vi "Init.vi"(8 "error in (no error)":errorcluster, 10 "Camera ID":string, 11 "ZWO_ASI in":refnum<class "ZWO_ASI.lvclass">) -> (0 "error out":errorcluster, 3 "ZWO_ASI out":refnum<class "ZWO_ASI.lvclass">)   [LabVIEW 2023, in "ZWO_ASI.lvlib" / "ZWO_ASI.lvclass"]
uses:
  ZWO_ASI.lvclass
  ZWO_ASI.lvclass/ZWO_ASI.ctl
  <userlib>/ASICamera2_no_err/ASICamera2_no_err.lvlib
  Interfaces/InitDeinitInterface/InitDeinitComm Messages/InitDone Msg/InitDone Msg.lvclass
  <vilib>/ActorFramework/Actor/Actor.lvclass
  typedefs/instrumentType.ctl
  typedefs/typedefs.lvlib
  Applications/National Instruments/LabVIEW 2023 64-bit/vi.lib/ActorFramework/Actor/Actor.lvclass
  Users/alexandrosspiliotis/Documents/LV_DAQ_Project/ConcreteClasses/ConcreteInstrumentClasses/CameraClasses/ZWO_ASI_LV/ZWO_ASI/ZWO_ASI.lvclass
  Users/alexandrosspiliotis/Documents/LV_DAQ_Project/Interfaces/AbstractInstrumentClasses/Cameras_LV/CameraInterface/CameraInterface.lvclass
  Users/alexandrosspiliotis/Documents/LV_DAQ_Project/Interfaces/InitDeinitInterface/InitDeinit/InitDeinit.lvclass
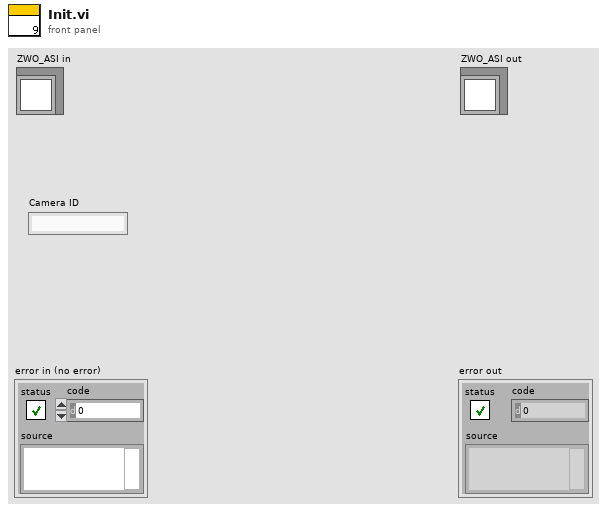
[diagram p1: front panel]
types:
  T1 = typedef "typedefs.lvlib/instrumentType.ctl" = enum16{"Spectrometer", "Camera", "Stepper"}
  T2 = cluster{"Name[0]":i8, "Name[1]":i8, "Name[2]":i8, "Name[3]":i8, "Name[4]":i8, "Name[5]":i8, "Name[6]":i8, "Name[7]":i8, "Name[8]":i8, "Name[9]":i8, "Name[10]":i8, "Name[11]":i8, "Name[12]":i8, "Name[13]":i8, "Name[14]":i8, "Name[15]":i8, "Name[16]":i8, "Name[17]":i8, "Name[18]":i8, "Name[19]":i8, "Name[20]":i8, "Name[21]":i8, "Name[22]":i8, "Name[23]":i8, "Name[24]":i8, "Name[25]":i8, "Name[26]":i8, "Name[27]":i8, "Name[28]":i8, "Name[29]":i8, "Name[30]":i8, "Name[31]":i8, "Name[32]":i8, "Name[33]":i8, "Name[34]":i8, "Name[35]":i8, "Name[36]":i8, "Name[37]":i8, "Name[38]":i8, "Name[39]":i8, "Name[40]":i8, "Name[41]":i8, "Name[42]":i8, "Name[43]":i8, "Name[44]":i8, "Name[45]":i8, "Name[46]":i8, "Name[47]":i8, "Name[48]":i8, "Name[49]":i8, "Name[50]":i8, "Name[51]":i8, "Name[52]":i8, "Name[53]":i8, "Name[54]":i8, "Name[55]":i8, "Name[56]":i8, "Name[57]":i8, "Name[58]":i8, "Name[59]":i8, "Name[60]":i8, "Name[61]":i8, "Name[62]":i8, "Name[63]":i8, "CameraID":i32, "MaxHeight":i32, "MaxWidth":i32, "IsColorCam":u32, "BayerPattern":u32, "SupportedBins[0]":i32, "SupportedBins[1]":i32, "SupportedBins[2]":i32, "SupportedBins[3]":i32, "SupportedBins[4]":i32, "SupportedBins[5]":i32, "SupportedBins[6]":i32, "SupportedBins[7]":i32, "SupportedBins[8]":i32, "SupportedBins[9]":i32, "SupportedBins[10]":i32, "SupportedBins[11]":i32, "SupportedBins[12]":i32, "SupportedBins[13]":i32, "SupportedBins[14]":i32, "SupportedBins[15]":i32, "SupportedVideoFormat[0]":u32, "SupportedVideoFormat[1]":u32, "SupportedVideoFormat[2]":u32, "SupportedVideoFormat[3]":u32, "SupportedVideoFormat[4]":u32, "SupportedVideoFormat[5]":u32, "SupportedVideoFormat[6]":u32, "SupportedVideoFormat[7]":u32, "@dummy control@":i8, "@dummy control@":i8, "@dummy control@":i8, "@dummy control@":i8, "PixelSize":dbl, "MechanicalShutter":u32, "ST4Port":u32, "IsCoolerCam":u32, "IsUSB3Host":u32, "IsUSB3Camera":u32, "ElecPerADU":sgl, "Unused[0]":i8, "Unused[1]":i8, "Unused[2]":i8, "Unused[3]":i8, "Unused[4]":i8, "Unused[5]":i8, "Unused[6]":i8, "Unused[7]":i8, "Unused[8]":i8, "Unused[9]":i8, "Unused[10]":i8, "Unused[11]":i8, "Unused[12]":i8, "Unused[13]":i8, "Unused[14]":i8, "Unused[15]":i8, "Unused[16]":i8, "Unused[17]":i8, "Unused[18]":i8, "Unused[19]":i8, "Unused[20]":i8, "Unused[21]":i8, "Unused[22]":i8, "Unused[23]":i8}
  T3 = typedef "typedefs.lvlib/InstrumentData.ctl" = cluster{"Instr Error":errorcluster, "Address":cluster{"address type":enum16{"VISA", "Index"}, "Address":string, "instrument type":T1}, "CurrentState":cluster{"Initialized":bool, "Connected":bool, "Running":bool, "Error":bool}, "Enqueuer":refnum<class "Message Enqueuer.lvclass">}
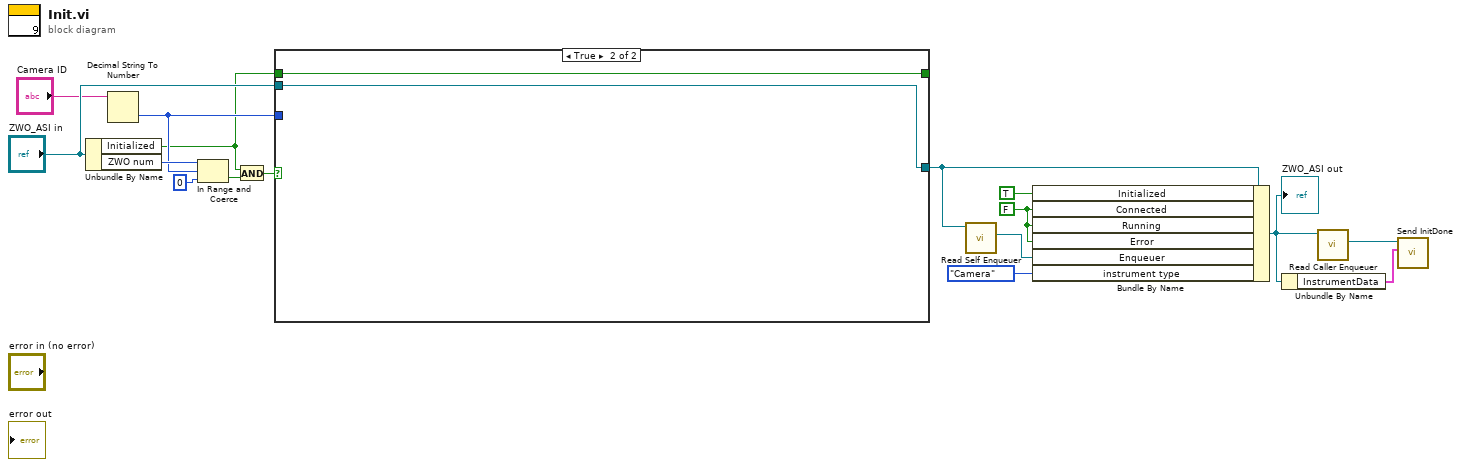
[diagram p0: block diagram]
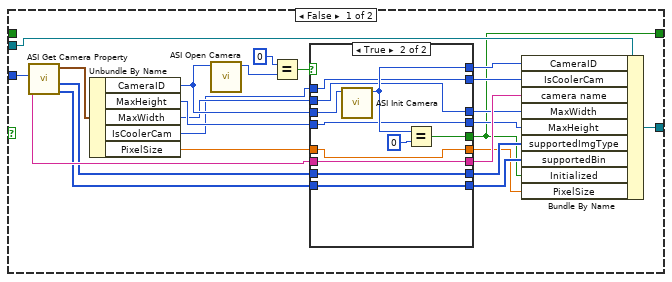
[diagram p2: hidden frame]
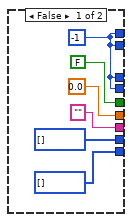
[diagram p3: hidden frame]
diagram:
  w6 = FALSE ("InstrumentData.CurrentState.Connected")
  n1 = Unbundle By Name("ZWO_ASI in") -> ("Initialized"=w8:bool, "ZWO num"=w14:i32)
  n2 = Decimal String To Number(string="Camera ID") -> (number=w10:i32)  [unwired: 2 in, 1 out]
  n3 = In Range and Coerce(upper limit=w14, x=w10, lower limit=0) -> (In Range?=w12:bool)  [unwired: 1 out]
  n4 = And(x=w8, y=w12) -> (x .and. y?=w11:bool)
  n5 = case shown="True" w11 {
    tunnel: w10 -> [w35 _]
    tunnel: "ZWO_ASI in" -> [w34 w58]
    tunnel: [w18 w59] -> _
    tunnel: w8 -> [_ w59]
    tunnel: [w17 w58] -> w2
    frame False {
      n6 = call <userlib>:"ASI Get Camera Property.vi"("iCameraIndex"=w35) -> ("supportedBin"=w27:i8[], "supportedImgType"=w26:i8[], "pASICameraInfo out"=w38:T2, "cameraName"=w31:string)  [unwired: 6 in, 1 out]
      n7 = Unbundle By Name(w38) -> ("CameraID"=w36:i32, "MaxHeight"=w29:i32, "MaxWidth"=w22:i32, "IsCoolerCam"=w21:u32, "PixelSize"=w20:dbl)
      n8 = call <userlib>:"ASI Open Camera.vi"("iCameraID"=w36) -> ("function return"=w40:i32)  [unwired: 10 in]
      n9 = Equal?(x=0, y=w40) -> (x = y?=w37:bool)
      n10 = case shown="True" w37 {
        tunnel: [FALSE w56] -> w18
        tunnel: w36 -> [_ w55]
        tunnel: [w45 w54] -> w33
        tunnel: [w45 w48] -> w32
        tunnel: w31 -> [_ w53]
        tunnel: ["" ("cameraName") w53] -> w30
        tunnel: w29 -> [_ w50]
        tunnel: [i8[] [] ("supportedBin") w52] -> w28
        tunnel: w27 -> [_ w52]
        tunnel: w26 -> [_ w51]
        tunnel: [i8[] [] ("supportedImgType") w51] -> w25
        tunnel: [w45 w50] -> w24
        tunnel: [w45 w49] -> w23
        tunnel: w22 -> [_ w49]
        tunnel: w21 -> [_ w48]
        tunnel: w20 -> [_ w47]
        tunnel: [0.0 ("PixelSize") w47] -> w19
        frame False {
          w45 = -1 ("function return")
        }
        frame True {
          n11 = call <userlib>:"ASI Init Camera.vi"("iCameraID"=w55) -> ("function return"=w54:i32)  [unwired: 10 in]
          n12 = Equal?(x=w54, y=0 ("x")) -> (x = y?=w56:bool)
        }
      }
      n13 = Bundle By Name(cluster=w34, "CameraID"=w33, "IsCoolerCam"=w32, "camera name"=w30, "MaxWidth"=w23, "MaxHeight"=w24, "supportedImgType"=w25, "supportedBin"=w28, "Initialized"=w18, "PixelSize"=w19) -> (w17:refnum<class "ZWO_ASI.lvclass">)
    }
    frame True {
    }
  }
  n14 = call <vilib>:"Read Self Enqueuer.vi"("Actor"=w2) -> ("Self Enqueuer"=w1:refnum<class "Message Enqueuer.lvclass">)  [unwired: 10 in]
  n15 = Bundle By Name(cluster=w2, "Initialized"=TRUE ("InstrumentData.CurrentState.Initialized"), "Connected"=w6, "Running"=w6, "Error"=w6, "Enqueuer"=w1, "instrument type"=instrumentType."Camera" ("InstrumentData.Address.instrument type")) -> (w5:refnum<class "ZWO_ASI.lvclass">)
  "ZWO_ASI out" <- w5
  n16 = Unbundle By Name(w5) -> ("InstrumentData"=w4:T3)
  n17 = call <vilib>:"Read Caller Enqueuer.vi"("Actor"=w5) -> ("Caller Enqueuer"=w9:refnum<class "Message Enqueuer.lvclass">)  [unwired: 10 in]
  n18 = call "Send InitDone.vi"("InstrumentData"=w4, "Message Enqueuer"=w9) -> ()  [unwired: 8 in, 2 out]
